vi "Flow.vi"() -> (1 "Flow (ml/min)":dbl format="%.2f")   [LabVIEW 2016]
uses:
  Kpro Globals.vi
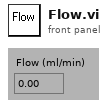
[diagram p1: front panel]
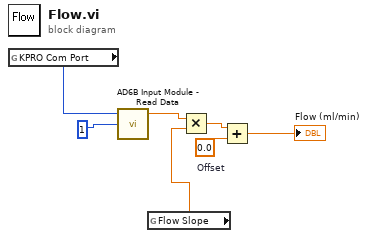
[diagram p0: block diagram]
diagram:
  w4 = 0.0  # Offset
  n1 = global read "Kpro Globals.vi" "KPRO Com Port"() -> (w2:i32)
  n2 = call "AD6B Input Module - Read Data.VI"("address (0 to 255)"=1, "port number (1:com2)"=w2) -> ("scaled data"=w6:dbl)  [unwired: 1 in, 2 out]
  n3 = global read "Kpro Globals.vi" "Flow Slope"() -> (w1:dbl)
  n4 = Multiply(x=w6, y=w1) -> (x*y=w5:dbl)
  n5 = Add(x=w5, y=w4) -> (x+y=→"Flow (ml/min)":dbl)
